vi "Initialize IAM Session.vi"(8 "error in (no error)":errorcluster, 11 "AWS Credentials":T1) -> (0 "error out":errorcluster, 3 "IAM Session":refnum<class "IAM Session.lvclass">)   [LabVIEW 2015, in "NI_AWS_IAM.lvlib" / "IAM Session.lvclass"]
uses:
  IAM Session.lvclass
  Core/HTTP Request/AWS Credentials.ctl
  Core/HTTP Request/Region.ctl
  Core/HTTP Request/HTTP Request.lvclass/HTTP Request.ctl
  Core/HTTP Request/Write Credentials.vi
  Core/HTTP Request/Write Region.vi
  Core/HTTP Request/Write Service.vi
  Core/HTTP Request/Write Verify Server.vi
  Core/HTTP Request/HTTP Request.lvclass
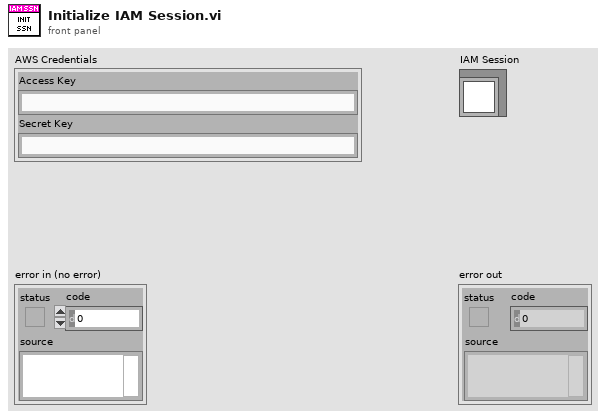
[diagram p1: front panel]
types:
  T1 = typedef "NI_AWS_Core.lvlib/HTTP Request.lvclass/AWS Credentials.ctl" = cluster{"Access Key":string, "Secret Key":string}
  T2 = typedef "NI_AWS_Core.lvlib/HTTP Request.lvclass/Region.ctl" = enum16{"us-east-1", "us-east-2", "us-west-1", "us-west-2", "ap-northeast-1", "ap-northeast-2", "ap-southeast-1", "ap-southeast-2", "ca-central-1", "eu-central-1", "eu-west-1", "eu-west-2", "sa-east-1"}
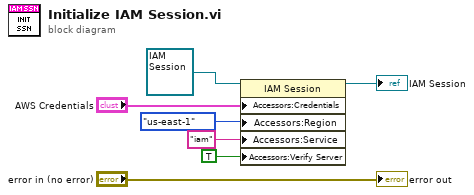
[diagram p0: block diagram]
diagram:
  n1 = property class="IAM Session"(reference=refnum<class "IAM Session.lvclass"> refnum ("NI_AWS_IAM.lvlib:IAM Session.lvclass"), "Accessors:Credentials"="AWS Credentials", "Accessors:Region"=Region."us-east-1" ("Region"), "Accessors:Service"="iam" ("Service"), "Accessors:Verify Server"=TRUE ("Verify Server")) -> (reference out=→"IAM Session":refnum<class "IAM Session.lvclass">)  [unwired: 1 in, 1 out]
  "error out" <- "error in (no error)"
